vi "TDMS AE.vi"(4 "Context":refnum<k7>, 7 "Control":T1=enum."Check Name", 8 "Error in":errorcluster, 9 "Channels":cluster{"Channel":string, "Data":dbl}[](array[cluster]), 10 "Group Name":string, 11 "Logging path":path) -> (0 "error out":errorcluster, 3 "Is Fname changed?":bool)   [LabVIEW 2021]
uses:
  TDMS States.ctl
  <vilib>/National Instruments/Asynchronous TDMS Logger/_Typedefs/Multiple Files Configuration.ctl
  <vilib>/National Instruments/Asynchronous TDMS Logger/_Typedefs/Multiple Files Action.ctl
  <vilib>/National Instruments/Asynchronous TDMS Logger/_Typedefs/Old Files Configuration.ctl
  <vilib>/National Instruments/Asynchronous TDMS Logger/_Typedefs/Folder Size Limit Reached.ctl
  <vilib>/National Instruments/Asynchronous TDMS Logger/TDMS Logger.lvclass
  72aef23a-740f-4946-8ab4-ac58cd915ab0.vi
  <vilib>/addons/TestStand/_TSUtility.llb/TestStand - Get Property Value (Number).vi
  <vilib>/National Instruments/Asynchronous TDMS Logger/API/Log Data DBL.vi
  <vilib>/National Instruments/Asynchronous TDMS Logger/API/Log Event.vi
  Display.lvlib
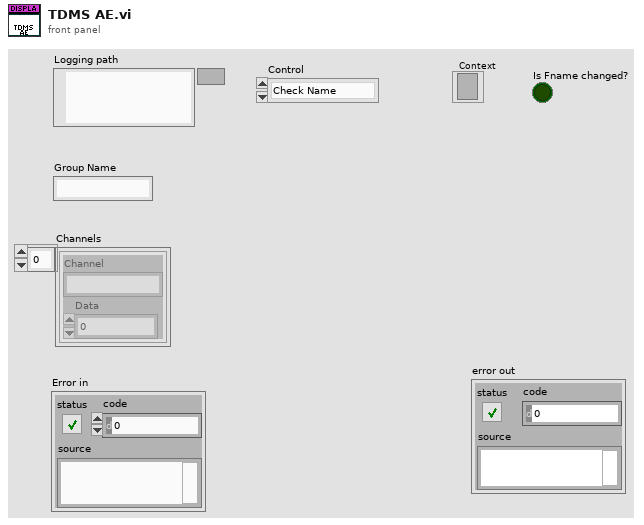
[diagram p1: front panel]
types:
  T1 = typedef "Display.lvlib/TDMS States.ctl" = enum16{"Open", "Write", "Check Name", "Stop"}
  T2 = typedef "TDMS Logger.lvlib/TDMS Logger.lvclass/Old Files Configuration.ctl" = cluster{"Action on Max Folder Size":T3, "Max # Files in Folder":i32}
  T3 = typedef "TDMS Logger.lvlib/TDMS Logger.lvclass/Folder Size Limit Reached.ctl" = enum16{"Do Nothing", "Remove Oldest Files"}
  T4 = typedef "TDMS Logger.lvlib/TDMS Logger.lvclass/Multiple Files Configuration.ctl" = cluster{"Multiple Files Action":T5, "Max File Size (MB)":dbl, "Max Time in File (s)":dbl}
  T5 = typedef "TDMS Logger.lvlib/TDMS Logger.lvclass/Multiple Files Action.ctl" = enum16{"Seperate based on size", "Seperate based on time", "Single file"}
  T6 = typedef "TDMS Logger.lvlib/TDMS Logger.lvclass/Logger Status Information.ctl" = cluster{"Number of Data Files":i32, "Current File Size (MB)":dbl, "Current Logs Path":path, "Last File Start":timestamp, "Throughput (MB/s)":dbl}
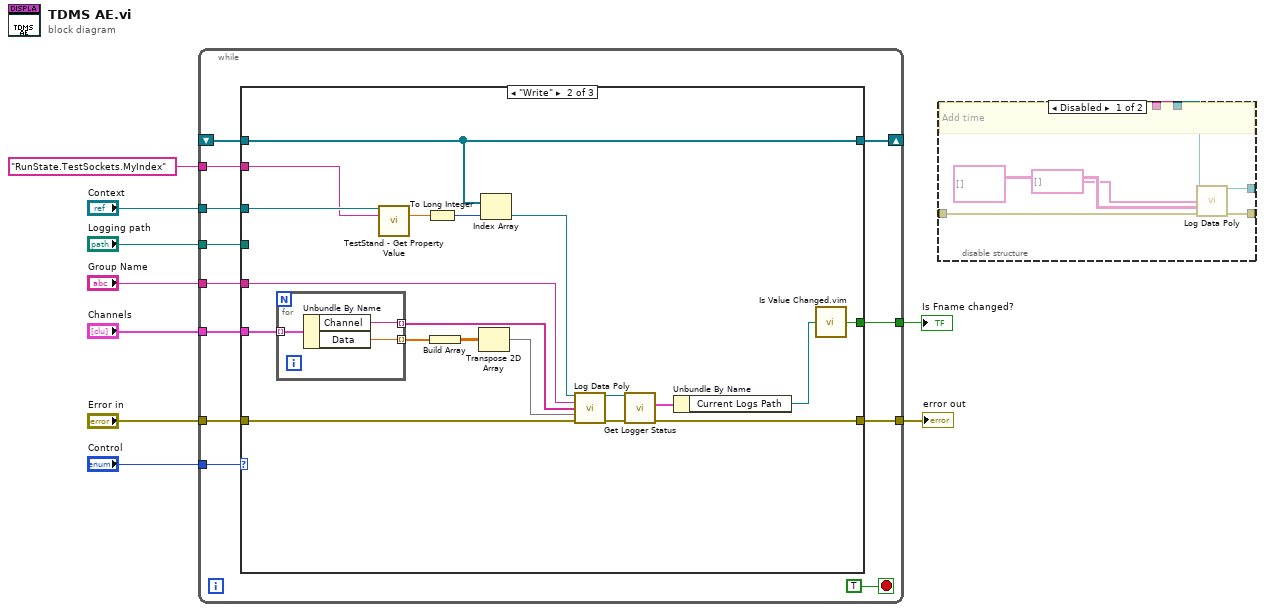
[diagram p0: block diagram]
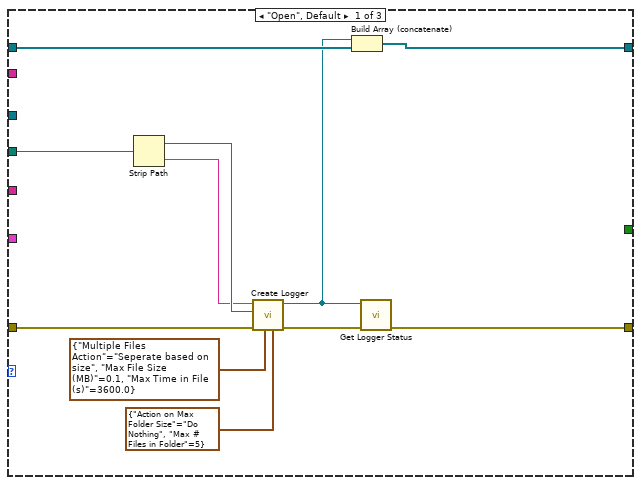
[diagram p2: hidden frame]
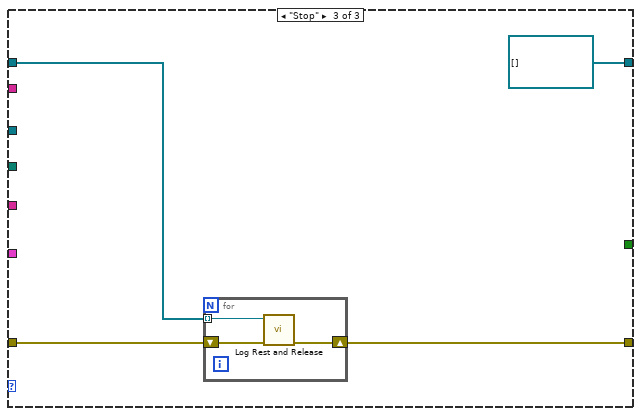
[diagram p3: hidden frame]
diagram:
  n1 = while {
    tunnel: [w21] -> w9
    tunnel: "Group Name" -> [w20]
    tunnel: "Channels" -> [w19]
    tunnel: "Context" -> [w18]
    tunnel: "Logging path" -> [w17]
    shift-right: [w15] -> _
    shift-left: _ -> [w14]
    tunnel: "Error in" -> [w13]
    tunnel: "Control" -> [w12]
    tunnel: [w11] -> w2
    tunnel: "RunState.TestSockets.MyIndex" ("Lookup String") -> [w10]
    stop <- TRUE stop-if-true
    n2 = case shown="\"Write\"" w12 {
      tunnel: [w30 w46 refnum<class "TDMS Logger.lvclass">[] []] -> w15
      tunnel: w14 -> [w25 w46 w57]
      tunnel: [w22 w37 w58] -> w21
      tunnel: w20 -> [_ w35 _]
      tunnel: w19 -> [_ w45 _]
      tunnel: w18 -> [_ w49 _]
      tunnel: w17 -> [w27 _ _]
      tunnel: w13 -> [w26 w36 w55]
      tunnel: [_ w38 _] -> w11
      tunnel: w10 -> [_ w33 _]
      frame "Open", Default {
        n3 = Strip Path(path=w27) -> (stripped path=w29:path, name=w28:string)
        n4 = call <vilib>:"Create Logger.vi"("Old Files Configuration"=T2 {"Action on Max Folder Size"=enum."Do Nothing", "Max # Files in Folder"=5}, "Multiple Files Configuration"=T4 {"Multiple Files Action"=enum."Seperate based on size", "Max File Size (MB)"=0.1, "Max Time in File (s)"=3600.0}, "Error In"=w26, "Base Folder"=w29, "Base File Name"=w28) -> ("Error Out"=w23:errorcluster, "TDMS Log Out"=w24:refnum<class "TDMS Logger.lvclass">)  [unwired: 4 in, 1 out]
        n5 = Build Array (concatenate)(w24, w25) -> (w30:refnum<class "TDMS Logger.lvclass">[])
        n6 = call <vilib>:"Get Logger Status.vi"("Error In"=w23, "TDMS Log In"=w24) -> ("Error Out"=w22:errorcluster)  [unwired: 6 in, 3 out]
      }
      frame "Write" {
        n7 = for {
          tunnel: w45 -> [w54] mode=indexing
          tunnel: [w52] -> w44 mode=indexing
          tunnel: [w53] -> w43 mode=indexing
          n8 = Unbundle By Name(w54) -> ("Channel"=w52:string, "Data"=w53:dbl)
        }
        n9 = call-poly <vilib>:"TestStand - Get Property Value.vi"("Sequence Context In"=w49, "Lookup String"=w33) -> ("Value"=w51:dbl)  [unwired: 11 in, 2 out]
        n10 = To Long Integer(number=w51) -> (32bit integer=w50:i32)
        n11 = Build Array(w43) -> (w48:dbl[][])
        n12 = Transpose 2D Array(2D array=w48) -> (transposed array=w47:dbl[][])
        n13 = Index Array(array=w46, index=w50) -> (element=w34:refnum<class "TDMS Logger.lvclass">)
        n14 = call-poly <vilib>:"Log Data Poly.vi"("TDMS Log In"=w34, "Group Name"=w35, "Channels Names"=w44, "DBL Data"=w47, "Error In"=w36) -> ("TDMS Log Out"=w41:refnum<class "TDMS Logger.lvclass">, "Error Out"=w42:errorcluster)  [unwired: 9 in]
        n15 = call <vilib>:"Get Logger Status.vi"("Error In"=w42, "TDMS Log In"=w41) -> ("Error Out"=w37:errorcluster, "Logger Status"=w40:T6)  [unwired: 6 in, 2 out]
        n16 = Unbundle By Name(w40) -> ("Current Logs Path"=w39:path)
        n17 = call "Is Value Changed.vim"("value"=w39) -> ("changed or first call?"=w38:bool)
      }
      frame "Stop" {
        n18 = for {
          shift-right: [w60] -> w58
          shift-left: w55 -> [w61]
          tunnel: w57 -> [w59] mode=indexing
          n19 = call <vilib>:"Log Rest and Release.vi"("Error In"=w61, "TDMS Log In"=w59) -> ("Error Out"=w60:errorcluster)  [unwired: 9 in]
        }
      }
    }
  }
  "error out" <- w9
  "Is Fname changed?" <- w2
  n20 = disable-structure shown="Disabled" {
    disable-tunnel: _ -> [w68 _]
    disable-tunnel: _ -> [w67 _]
    disable-tunnel: [w66 _] -> _
    disable-tunnel: _ -> [w64 _]
    disable-tunnel: [w63 _] -> _
    frame Disabled {
      # "Add time"
      n21 = call-poly <vilib>:"Log Data Poly.vi"("TDMS Log In"=w68, "Group Name (Events)"=w64, "Channels Names"=string[] [], "String Data"=string[][] [], "Error In"=w67) -> ("TDMS Log Out"=w63:refnum<class "TDMS Logger.lvclass">, "Error Out"=w66:errorcluster)  [unwired: 9 in]
    }
    frame Enabled {
    }
  }
